vi "NanotecSMCPD.get resources.vi"(0 "i ref in":refnum<vi>, 2 "axisNumber":i32, 5 "error in (no error)":errorcluster) -> (14 "i ref out":refnum<vi>, 16 "VISA resource":refnum<visa-resource-name>, 17 "address":i32, 19 "error out":errorcluster)   [LabVIEW 2014, in "NanotecSMCPD.lvlib"]
doc: "Gets the resources (VISA, address) for the specified axis."
uses:
  NanotecSMCPD.lvlib
  CS_Core/CSSystem/CoreDefs/CoreDefs.error_type.ctl
  CS_Core/CSSystem/CoreDefs/CoreDefs.error_severity.ctl
  CS_Core/CSApplicationBaseClasses/MotorBase/MotorBase.lvlib
  CS_Core/CSSystem/CoreLib/CoreLib.lvlib
  CS_Core/BaseProcess/BaseProcess.lvlib
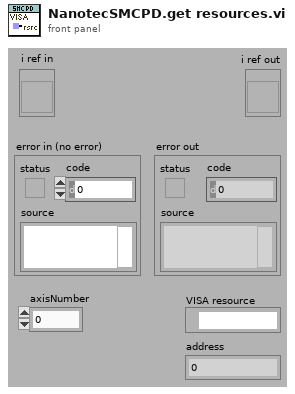
[diagram p1: front panel]
types:
  T1 = typedef "CoreDefs.error_severity.ctl" = enum16{"undefined", "information", "warning", "error", "fatal"}
  T2 = typedef "CoreDefs.error_type.ctl" = enum16{"no error", "can't load process", "can't unload process", "process does not exist", "can't install process", "can't remove process", "unknown function", "time out", "can't execute function", "duplicate queue name", "super not found", "caller queue invalid", "can't ping process", "unknown error", "VISA Error", "VISA timeout", "GPIB timeout", "GPIB error", "communication error", "data type mismatch", "can't read data from OPC server", "can't write data to OPC server", "OET error", "function not implemented", "process already exists", "invalid Shared Variable name", "error writing Shared Variable", "error reading Shared Variable", "invalid client name", "corrupt database", "unknown class", "call not authorized", "parameter out of range", "OET timeout: can't get data to modify", "invalid queue name", "requested operation incompatible with current state", "event undefined", "event disabled", "state undefined", "caller is not a friend", "EventBuilder: bad eventID", "EventBuilder: no DAQ devices", "a thread must not stop itself", "UNUSED ELEMENT4", "DiscArchiver: eventData incomplete", "DiscArchiver: eventData does not belong to run", "DiscArchiver: can't open file", "DiscArchiver: can't write to file", "DiscArchiver: available disc space low", "can't acquire semaphore", "error reading data from database", "notifier object is not existing", "can't register process", "can't unregister process", "illegal event type", "object disabled", "object already exists", "can't change state", "Instrument not found", "no connection to remote node", "invalid reference", "N/A", "UNUSED ELEMENT 1", "element not found", "illegal TCP/IP connection detected", "object does not exist", "invalid access ID", "unknown CS system", "invalid privilige", "unsupported data type", "unsupported server type", "IO server already exists", "Shared Variable already exists"}
  T3 = typedef "BaseProcess.lvlib/BaseProcess.i attribute.ctl" = cluster{"EventStatus":string, "EventError":i32, "PresetEvtWatchD":i32, "PresetPdcWatchD":i32, "EventTimeout":i32, "PeriodicInterval":i32, "Interface":string[], "Address":string[], "Special":string[], "PeriodicError":i32, "PeriodicStatus":string, "SuperProc":string, "Descriptors":T4[], "CaseRef":refnum<vi>, "PdcRef":refnum<vi>, "Thread Ref":refnum<vi>, "eventErrorID":i32, "eventStatusID":i32, "periodicErrorID":i32, "periodicStatusID":i32, "pdcCtrID":i32}
  T4 = typedef "BaseProcess.lvlib/BaseProcess.descriptor definition.ctl" = cluster{"selector":string, "descriptor":T5}
  T5 = typedef "BaseProcess.lvlib/BaseProcess.descriptor string definition.ctl" = string
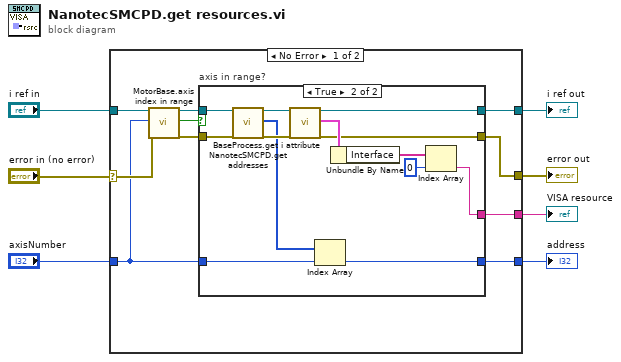
[diagram p0: block diagram]
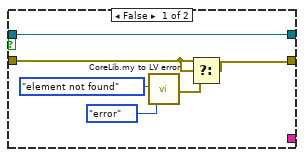
[diagram p2: hidden frame]
diagram:
  n1 = case shown="No Error" "error in (no error)" {
    selector: "error in (no error)" -> [w12 w37]
    tunnel: "i ref in" -> [w17 w38]
    tunnel: [w13 w38] -> w6
    tunnel: [w9 w37] -> w5
    tunnel: [w10 _] -> w4
    tunnel: "axisNumber" -> [w11 _]
    tunnel: [w8 _] -> w1
    frame No Error {
      n2 = call "MotorBase.axis index in range.vi"("i ref in"=w17, "axisIndex"=w11, "error in (no error)"=w12) -> ("i ref out"=w14:refnum<vi>, "in range"=w16:bool, "error out"=w15:errorcluster)  [unwired: 14 in]
      n3 = case "axis in range?" shown="True" w16 {
        tunnel: w15 -> [w20 w34]
        tunnel: [w19 w28] -> w9
        tunnel: [w18 w29] -> w13
        tunnel: w14 -> [w18 w35]
        tunnel: w11 -> [_ w30]
        tunnel: [_ w25] -> w10
        tunnel: [_ w24] -> w8
        frame False {
          n4 = call "CoreLib.my to LV error.vi"("ErrorTypes"=CoreDefs.error_type."element not found", "severityLevel"=CoreDefs.error_severity."error") -> ("myErrorCluster"=w23:errorcluster)  [unwired: 16 in, 1 out]
          n5 = Select(t=w20, s=w20, f=w23) -> (s? t:f=w19:errorcluster)
        }
        frame True {
          n6 = call "NanotecSMCPD.get addresses.vi"("i ref in"=w35, "error in (no error)"=w34) -> ("i ref out"=w33:refnum<vi>, "controllerAddresses"=w31:i32[], "error out"=w32:errorcluster)  [unwired: 15 in]
          n7 = call "BaseProcess.get i attribute.vi"("i ref in"=w33, "error in (no error)"=w32) -> ("i ref out"=w29:refnum<vi>, "i attribute"=w36:T3, "error out"=w28:errorcluster)  [unwired: 15 in]
          n8 = Index Array(array=w31, index=w30) -> (element=w24:i32)
          n9 = Unbundle By Name(w36) -> ("Interface"=w27:string[])
          n10 = Index Array(array=w27, index=0) -> (element=w25:string)
        }
      }
    }
    frame Error {
    }
  }
  "error out" <- w5
  "i ref out" <- w6
  "VISA resource" <- w4
  "address" <- w1
